vi "DragDeltaVelocity.vi"(3 "Drag dV":dbl, 10 "Robot Velocity":dbl, 11 "Drag Coefficients":dbl) -> ()   [LabVIEW 2012]
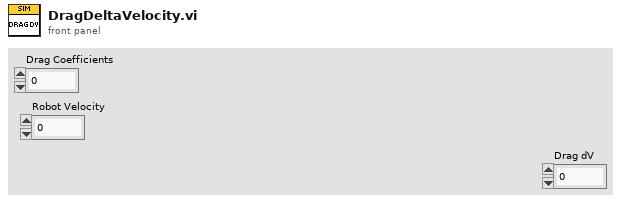
[diagram p1: front panel]
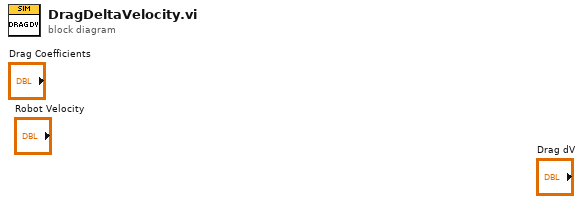
[diagram p0: block diagram]
diagram:
